vi "Get Device Config.vi"() -> (3 "value":i32)   [LabVIEW 2019, in "ESP301.lvlib"]
uses:
  ESP301.lvlib
  <vilib>/Utility/config.llb/Read Key (I32).vi
  <vilib>/Utility/config.llb/NI_LVConfig.lvlib
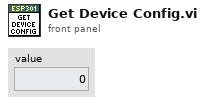
[diagram p1: front panel]
types:
  T1 = typedef "NI_LVConfig.lvlib/Config Data RefNum.ctl" = refnum<k1>
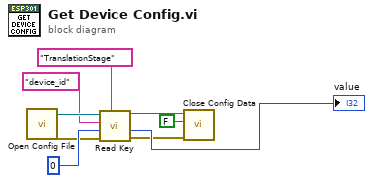
[diagram p0: block diagram]
diagram:
  n1 = call "Open Config File.vi"() -> ("error out"=w6:errorcluster, "Refnum out"=w7:T1)  [unwired: 10 in]
  n2 = call-poly <vilib>:"Read Key.vi"("section"="TranslationStage", "error in (no error)"=w6, "default value"=0, "key"="device_id", "refnum"=w7) -> ("error out"=w3:errorcluster, "value"=→"value":i32, "refnum out"=w2:T1)  [unwired: 3 in, 1 out]
  n3 = call <vilib>:"Close Config Data.vi"("error in (no error)"=w3, "write file if changed (T)"=FALSE, "refnum"=w2) -> ()  [unwired: 7 in, 2 out]
